vi "Autonomous Independent.vi"() -> ()   [LabVIEW 2013]
doc: "This VI is called when autonomous begins, and will automatically be terminated when autonomous ends. You can carry out timed or sensor driven robot movement independently without needing to return to the caller."
uses:
  Robot Global Data.vi
  <vilib>/Rock Robotics/WPI/SafetyOutput/WPI_SafetyOutputConfigMenu.ctl
panel:
  in  "Shooter timer":u32=500
  in  "1st Distance":dbl=-3400.0
  # "Be sure to right-click and choose Data Operations>>Make Current Value default if you want to save the array values with the VI"
  # "pra frente negativo\npra tras positivo"
  # "-3200"
  # "500"
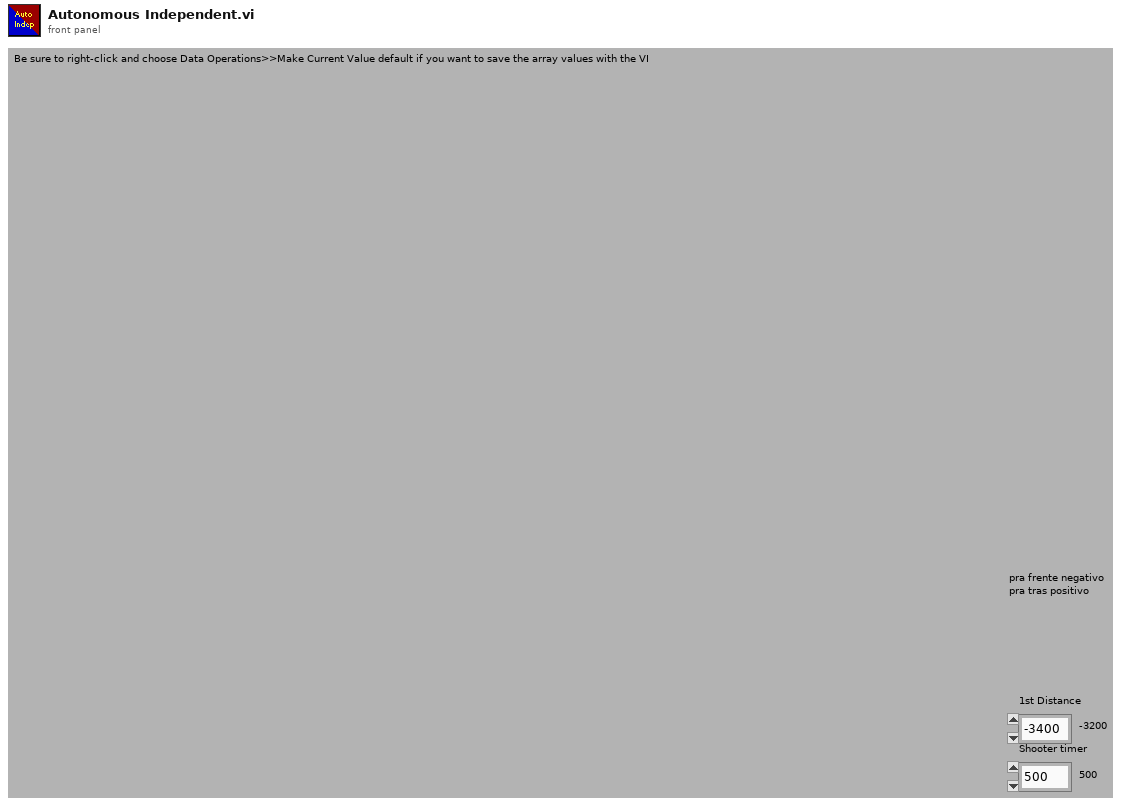
[diagram p1: front panel]
types:
  T1 = typedef "WPI_SafetyOutputConfigMenu.ctl" = enum16{"Enable", "Disable"}
  T2 = typedef "WPI_RobotDriveDevRef.ctl" = cluster{"DevStatus":errorcluster, "Motors[]":T3[], "Square Inputs":bool, "Max Output":dbl, "Isochronous":bool}
  T3 = typedef "WPI_MotorControlDeviceRef.ctl" = cluster{"DeviceStatus":errorcluster, "Type":enum16{"PWM", "CAN"}, "PWM":cluster{"Digital Module":T4, "PWM Channel":T5, "DeadBand":T6}, "CAN":cluster{"Device Number":u8, "Control Mode":T7, "Semaphore":T8, "Max Vout":dbl}, "Invert":bool, "TransformRef":T9, "InvTransformRef":T9}
  T4 = typedef "FPGA_TypedefDigitalModule.ctl" = enum16{"Digital Module 1", "Digital Module 2"}
  T5 = typedef "FPGA_DIOPWMChannel.ctl" = enum8{"PWM 1", "PWM 2", "PWM 3", "PWM 4", "PWM 5", "PWM 6", "PWM 7", "PWM 8", "PWM 9", "PWM 10", "Invalid"}
  T6 = typedef "WPI_PWMDeadband.ctl" = cluster{"Name":string, "maxPositivePwm":i32, "minPositivePwm":i32, "centerPwm":i32, "maxNegativePwm":i32, "minNegativePwm":i32, "angularRange":u16}
  T7 = typedef "WPI_CANJaguar_ControlMode.ctl" = enum8{"Percent VBus", "Current", "Speed", "Position", "Voltage"}
  T8 = typedef "Semaphore RefNum" = refnum<k1>
  T9 = typedef "WPI_PWMTransform_ConPane.ctl" = refnum<vi>
  T10 = typedef "WPI_EncoderDevRef.ctl" = cluster{"DevStatus":errorcluster, "EncoderIndex":T11, "CounterIndex":T12, "DistancePerCount":dbl, "Decoding Type":T13}
  T11 = typedef "FPGA_EncoderIdx.ctl" = enum8{"Enc 0", "Enc 1", "Enc 2", "Enc 3", "Invalid"}
  T12 = typedef "FPGA_CounterCtrSystemIndex.ctl" = enum8{"Ctr 0", "Ctr 1", "Ctr 2", "Ctr 3", "Ctr 4", "Ctr 5", "Ctr 6", "Ctr 7", "Invalid"}
  T13 = typedef "WPI_EncoderType.ctl" = enum16{"1x", "2x", "4x"}
  T14 = typedef "WPI_ServoDeviceRef.ctl" = cluster{"DeviceStatus":errorcluster, "Digital Module":T4, "PWM Channel":T5, "DeadBand":T6}
  T15 = typedef "WPI_DigitalInputDevRef.ctl" = cluster{"DevStatus":errorcluster, "DIO Channel":T16, "Digital Module":T4}
  T16 = typedef "FPGA_DIOChannel.ctl" = enum8{"DIO 1", "DIO 2", "DIO 3", "DIO 4", "DIO 5", "DIO 6", "DIO 7", "DIO 8", "DIO 9", "DIO 10", "DIO 11", "DIO 12", "DIO 13", "DIO 14", "Invalid"}
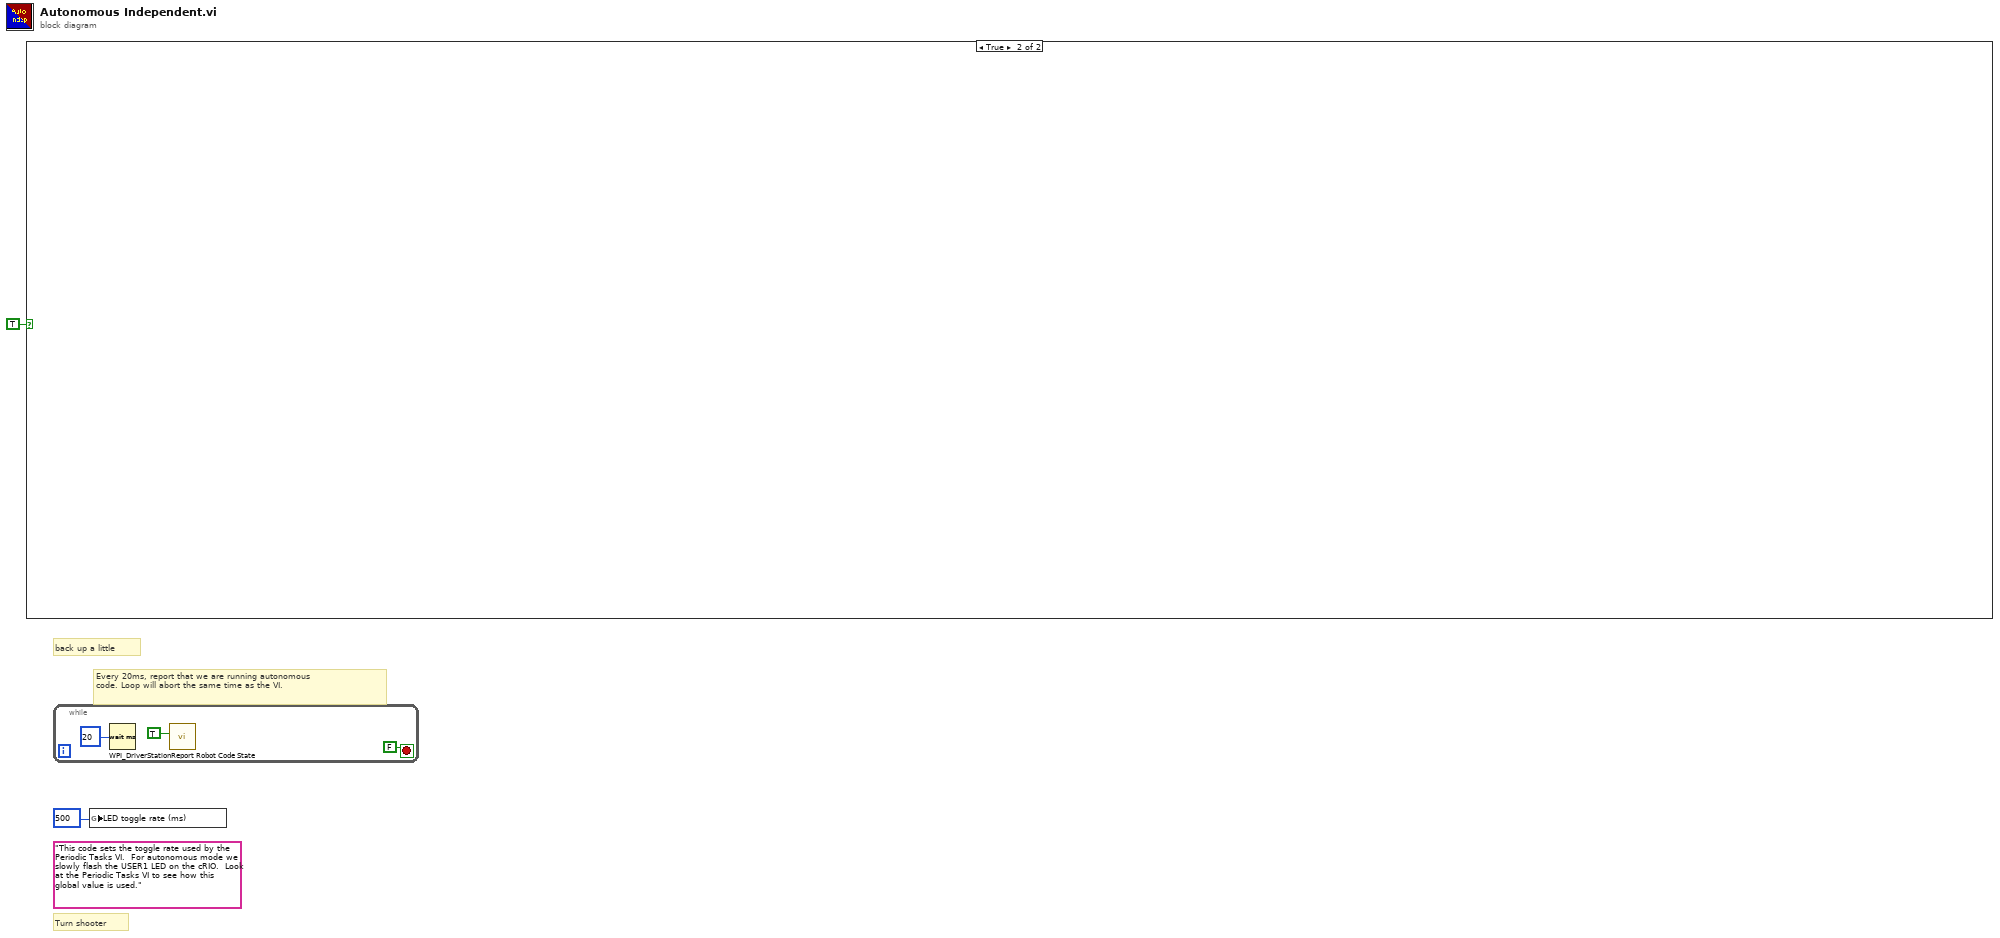
[diagram p0: block diagram]
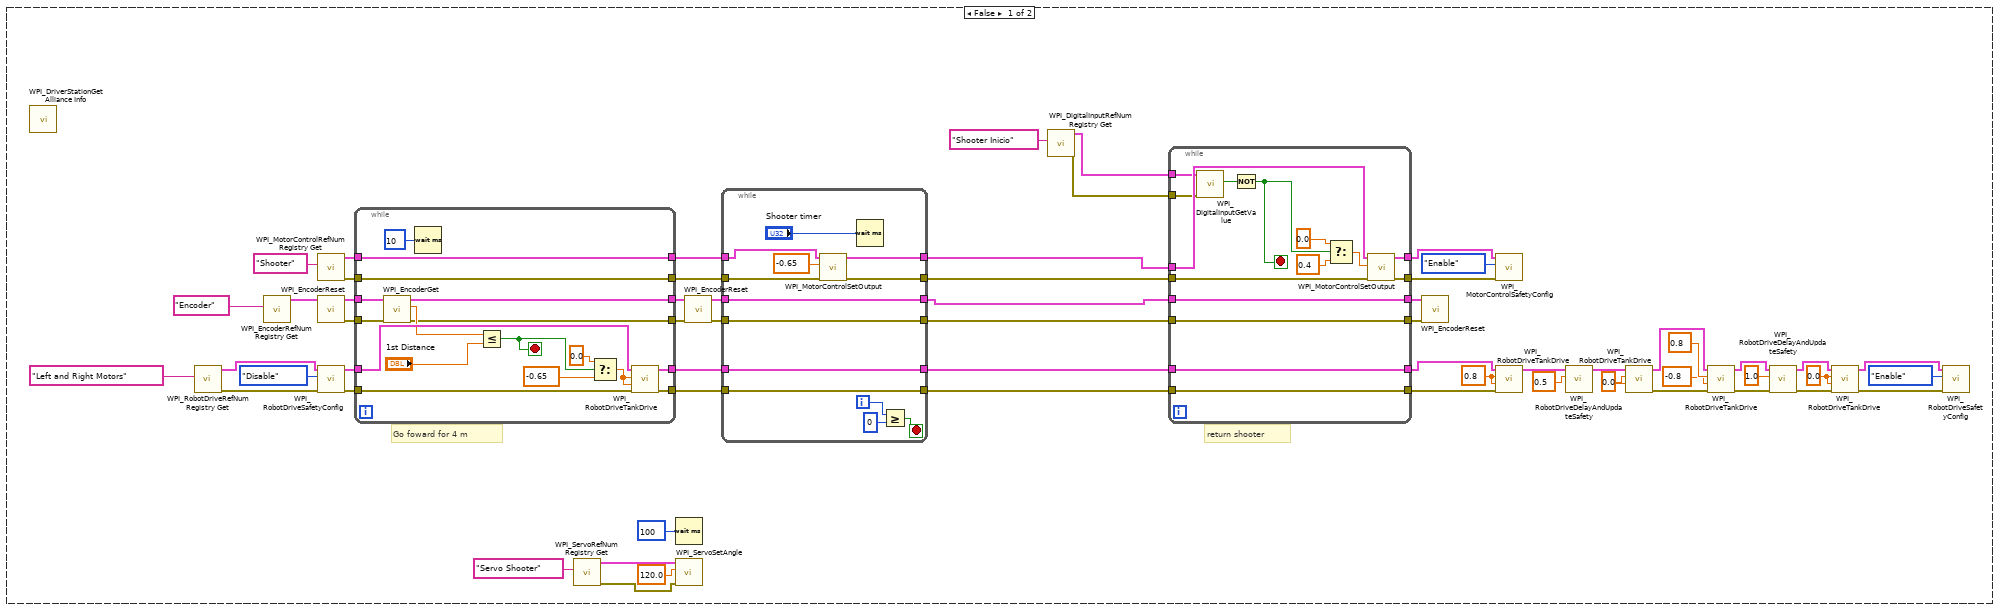
[diagram p2: hidden frame]
diagram:
  (unwired) "This code sets the toggle rate used by the Periodic Tasks VI.  For autonomous mode we slowly flash the USER1 LED on the cRIO.  Look at the Periodic Tasks VI to see how this global value is used."
  # "Turn shooter"
  # "back up a little"
  # "Every 20ms, report that we are running autonomous\ncode. Loop will abort the same time as the VI."
  n1 = case shown="True" TRUE {
    frame False {
      w27 = 0.0 ("f")
      w37 = 0.0 ("f")
      w36 = 0.8 ("f")
      # "return shooter"
      # "Go foward for 4 m"
      n2 = call <vilib>:"WPI_DriverStationGet Alliance Info.vi"() -> ()  [unwired: 12 out]
      n3 = call <vilib>:"WPI_RobotDriveRefNum Registry Get.vi"("refnum name"="Left and Right Motors") -> ("error out"=w56:errorcluster, "RobotDriveDevRef"=w55:T2)  [unwired: 9 in]
      n4 = call <vilib>:"WPI_EncoderRefNum Registry Get.vi"("refnum name"="Encoder") -> ("EncoderDevRef"=w61:T10)  [unwired: 9 in, 1 out]
      n5 = call <vilib>:"WPI_MotorControlRefNum Registry Get.vi"("refnum name"="Shooter") -> ("error out"=w50:errorcluster, "MotorControlDevRef"=w51:T3)  [unwired: 9 in]
      n6 = call <vilib>:"WPI_EncoderReset.vi"("EncoderDevRef"=w61) -> ("error out"=w58:errorcluster, "EncoderDevRef"=w59:T10)  [unwired: 9 in]
      n7 = call <vilib>:"WPI_RobotDriveSafetyConfig.vi"("error in (no error)"=w56, "mode"=WPI_SafetyOutputConfigMenu."Disable", "RobotDriveDevRef"=w55) -> ("error out"=w52:errorcluster, "RobotDriveDevRef"=w53:T2)  [unwired: 7 in]
      n8 = while {
        tunnel: w59 -> [w104]
        tunnel: w58 -> [w105]
        tunnel: w53 -> [w107]
        tunnel: w52 -> [w106]
        tunnel: [w96] -> w43
        tunnel: w51 -> [w96]
        tunnel: [w95] -> w42
        tunnel: w50 -> [w95]
        tunnel: [w94] -> w39
        tunnel: [w93] -> w38
        tunnel: [w92] -> w49
        tunnel: [w91] -> w48
        stop <- w98 stop-if-true
        n9 = call <vilib>:"WPI_EncoderGet.vi"("error in (no error)"=w105, "EncoderDevRef"=w104) -> ("error out"=w91:errorcluster, "Distance"=w103:dbl, "EncoderDevRef"=w92:T10)  [unwired: 4 in, 3 out]
        n10 = Wait (ms)(milliseconds to wait=u32 10) -> ()  [unwired: 1 out]
        n11 = Less Or Equal?(x=w103, y="1st Distance") -> (x <= y?=w98:bool)
        n12 = Select(t=0.0, s=w98, f=-0.65) -> (s? t:f=w99:dbl)
        n13 = call <vilib>:"WPI_RobotDriveTankDrive.vi"("error in (no error)"=w106, "Right axis value"=w99, "Left axis value"=w99, "RobotDriveDevRef"=w107) -> ("error out"=w93:errorcluster, "RobotDriveDevRef"=w94:T2)  [unwired: 5 in, 1 out]
      }
      n14 = call <vilib>:"WPI_ServoRefNum Registry Get.vi"("refnum name"="Servo Shooter") -> ("error out"=w12:errorcluster, "ServoDeviceRef"=w13:T14)  [unwired: 9 in]
      n15 = Wait (ms)(milliseconds to wait=u32 100) -> ()  [unwired: 1 out]
      n16 = call <vilib>:"WPI_ServoSetAngle.vi"("error in (no error)"=w12, "Angle"=120.0 ("t"), "ServoDeviceRef"=w13) -> ()  [unwired: 7 in, 2 out]
      n17 = call <vilib>:"WPI_EncoderReset.vi"("error in (no error)"=w48, "EncoderDevRef"=w49) -> ("error out"=w40:errorcluster, "EncoderDevRef"=w41:T10)  [unwired: 8 in]
      n18 = while {
        tunnel: w43 -> [w70]
        tunnel: w42 -> [w69]
        tunnel: [w68] -> w11
        tunnel: w41 -> [w64]
        tunnel: [w67] -> w8
        tunnel: w40 -> [w67]
        tunnel: [w66] -> w7
        tunnel: w39 -> [w66]
        tunnel: w38 -> [w63]
        tunnel: [w65] -> w10
        tunnel: [w64] -> w9
        tunnel: [w63] -> w6
        i -> [w75]
        stop <- w73 stop-if-true
        n19 = call <vilib>:"WPI_MotorControlSetOutput.vi"("error in (no error)"=w69, "Output"=-0.65 ("f"), "MotorControlDevRef"=w70) -> ("error out"=w65:errorcluster, "MotorControlDevRef"=w68:T3)  [unwired: 6 in, 1 out]
        n20 = Wait (ms)(milliseconds to wait="Shooter timer") -> ()  [unwired: 1 out]
        n21 = Greater Or Equal?(x=w75, y=0) -> (x >= y?=w73:bool)
      }
      n22 = call <vilib>:"WPI_DigitalInputRefNum Registry Get.vi"("refnum name"="Shooter Inicio") -> ("error out"=w3:errorcluster, "DigitalInputDevRef"=w4:T15)  [unwired: 9 in]
      n23 = while {
        tunnel: w11 -> [w90]
        tunnel: w10 -> [w89]
        tunnel: w6 -> [w84]
        tunnel: [w78] -> w35
        tunnel: [w84] -> w34
        tunnel: [w83] -> w46
        tunnel: [w82] -> w45
        tunnel: w9 -> [w80]
        tunnel: [w80] -> w30
        tunnel: w8 -> [w79]
        tunnel: [w79] -> w29
        tunnel: w7 -> [w78]
        tunnel: w4 -> [w77]
        tunnel: w3 -> [w76]
        stop <- w86 stop-if-true
        n24 = call <vilib>:"WPI_DigitalInputGetValue.vi"("error in (no error)"=w76, "DigitalInputDevRef"=w77) -> ("Value"=w85:bool)  [unwired: 7 in, 2 out]
        n25 = Not(x=w85) -> (.not. x?=w86:bool)
        n26 = Select(t=0.0, s=w86, f=0.4) -> (s? t:f=w88:dbl)
        n27 = call <vilib>:"WPI_MotorControlSetOutput.vi"("error in (no error)"=w89, "Output"=w88, "MotorControlDevRef"=w90) -> ("error out"=w82:errorcluster, "MotorControlDevRef"=w83:T3)  [unwired: 6 in, 1 out]
      }
      n28 = call <vilib>:"WPI_EncoderReset.vi"("error in (no error)"=w29, "EncoderDevRef"=w30) -> ()  [unwired: 8 in, 2 out]
      n29 = call <vilib>:"WPI_MotorControlSafetyConfig.vi"("error in (no error)"=w45, "mode"=WPI_SafetyOutputConfigMenu."Enable", "MotorControlDevRef"=w46) -> ()  [unwired: 7 in, 2 out]
      n30 = call <vilib>:"WPI_RobotDriveTankDrive.vi"("error in (no error)"=w34, "Right axis value"=w36, "Left axis value"=w36, "RobotDriveDevRef"=w35) -> ("RobotDriveDevRef"=w33:T2)  [unwired: 5 in, 2 out]
      n31 = call <vilib>:"WPI_RobotDriveDelayAndUpdateSafety.vi"("Delay (s)"=0.5, "RobotDriveDevRef"=w33) -> ("RobotDriveDevRef 2"=w31:T2)  [unwired: 8 in, 1 out]
      n32 = call <vilib>:"WPI_RobotDriveTankDrive.vi"("Right axis value"=w37, "Left axis value"=w37, "RobotDriveDevRef"=w31) -> ("error out"=w23:errorcluster, "RobotDriveDevRef"=w24:T2)  [unwired: 6 in, 1 out]
      n33 = call <vilib>:"WPI_RobotDriveTankDrive.vi"("error in (no error)"=w23, "Right axis value"=-0.8 ("Delay (s)"), "Left axis value"=0.8 ("Delay (s)"), "RobotDriveDevRef"=w24) -> ("error out"=w21:errorcluster, "RobotDriveDevRef"=w22:T2)  [unwired: 5 in, 1 out]
      n34 = call <vilib>:"WPI_RobotDriveDelayAndUpdateSafety.vi"("error in (no error)"=w21, "Delay (s)"=1.0, "RobotDriveDevRef"=w22) -> ("error out"=w25:errorcluster, "RobotDriveDevRef 2"=w26:T2)  [unwired: 7 in]
      n35 = call <vilib>:"WPI_RobotDriveTankDrive.vi"("error in (no error)"=w25, "Right axis value"=w27, "Left axis value"=w27, "RobotDriveDevRef"=w26) -> ("error out"=w17:errorcluster, "RobotDriveDevRef"=w18:T2)  [unwired: 5 in, 1 out]
      n36 = call <vilib>:"WPI_RobotDriveSafetyConfig.vi"("error in (no error)"=w17, "mode"=WPI_SafetyOutputConfigMenu."Enable", "RobotDriveDevRef"=w18) -> ()  [unwired: 7 in, 2 out]
    }
    frame True {
    }
  }
  n37 = while {
    stop <- FALSE stop-if-true
    n38 = Wait (ms)(milliseconds to wait=u32 20) -> ()  [unwired: 1 out]
    n39 = call <vilib>:"WPI_DriverStationReport Robot Code State.vi"("Autonomous"=TRUE) -> ()  [unwired: 10 in, 1 out]
  }
  n40 = global write "Robot Global Data.vi" "LED toggle rate (ms)"(u32 500 ("LED ms toggle rate")) -> ()
